vi "TAT_Start.vi"(8 "error In":errorcluster) -> (0 "error out":errorcluster)   [LabVIEW 2017]
uses:
  <vilib>/Utility/error.llb/DialogType.ctl
  Controls/Ass. Loop Control.ctl
  <vilib>/addons/database/Connection.llb/Conn ObjectReference.ctl
  2ffc4e95-467e-4723-8c12-a792954531b5.vi
  8539105e-fe5f-4c29-a376-e00596b22cdb.vi
  <vilib>/addons/database/Connection.llb/DB Tools Open Connec (Path).vi
  Global/Global 1.vi
  <vilib>/Instr/_visa.llb/VISA Configure Serial Port (Instr).vi
  <vilib>/addons/database/NI_Database_API.lvlib
  <vilib>/Utility/config.llb/NI_LVConfig.lvlib
panel:
  out "Para Value":T1
  out "PREVIOUS BARCODE":string
  out "PACKAGED QUANTITY":string
  out "SCANNED QUANTITY":string
  out "PACKAGE STICKER":string
  out "PRN to Print":string
  out "CYCLE RESULT:-":bool caption="LEAK RESULT:-"
  out "CYCLE STATUS STATION 2":string caption="CYCLE STATUS 2:-"
  out "SERIAL NO.:- 2":dbl
  in  "Model Selection:-":string(combo)
  out "CYCLE TIME:-":u32
  out "BARCODE STATION 2":string caption="QR CODE :-"
  out "CYCLE START:-":bool caption="LEAK RESULT:-"
  out "PREVIOUS BARCODE":string[](array[string])
  out "scanned":string
  out "Scanned Qty  2":string
  out "PROJECT :-":string
  out "PACKAGE Qty":string
  out "TORISHI CODE:-":string
  out "PART No.:-":string
  out "PLC STATUS:-":bool
  in  "Stop":bool
  out "QR STATION 1":string caption="QR CODE:-"
  out "RESULT STATION 1":bool caption="FINAL RESULT:-"
  out "USER:-":string
  out "PART NAME :-":string
  in  "ASS-Alarms":bool
  out "CYCLE STATUS STATION 1":string caption="CYCLE STATUS 1:-"
  out "DATE/TIME":string
  # "KAPSE SONS ROBOTICS\n& AUTOMATION"
  # "MODEL SELECTION:-"
  # "MIN"
  # "MAX"
  # "ACTUAL"
  # "STATUS"
  # "BLINKER CURRENT (mA)"
  # "POWER FOLD CURRENT (mA)"
  # "Nm"
  # "GLASS ACTUATOR CURRENT-1 (mA)"
  # "GLASS ACTUATOR CURRENT-2 (mA)"
  # "GROUND (Deg)"
  # "SKY (Deg)"
  # "EXTERIOR (Deg)"
  # "INTERIOR (Deg)"
  # "GLASS PULL OUT LOAD (Kg)"
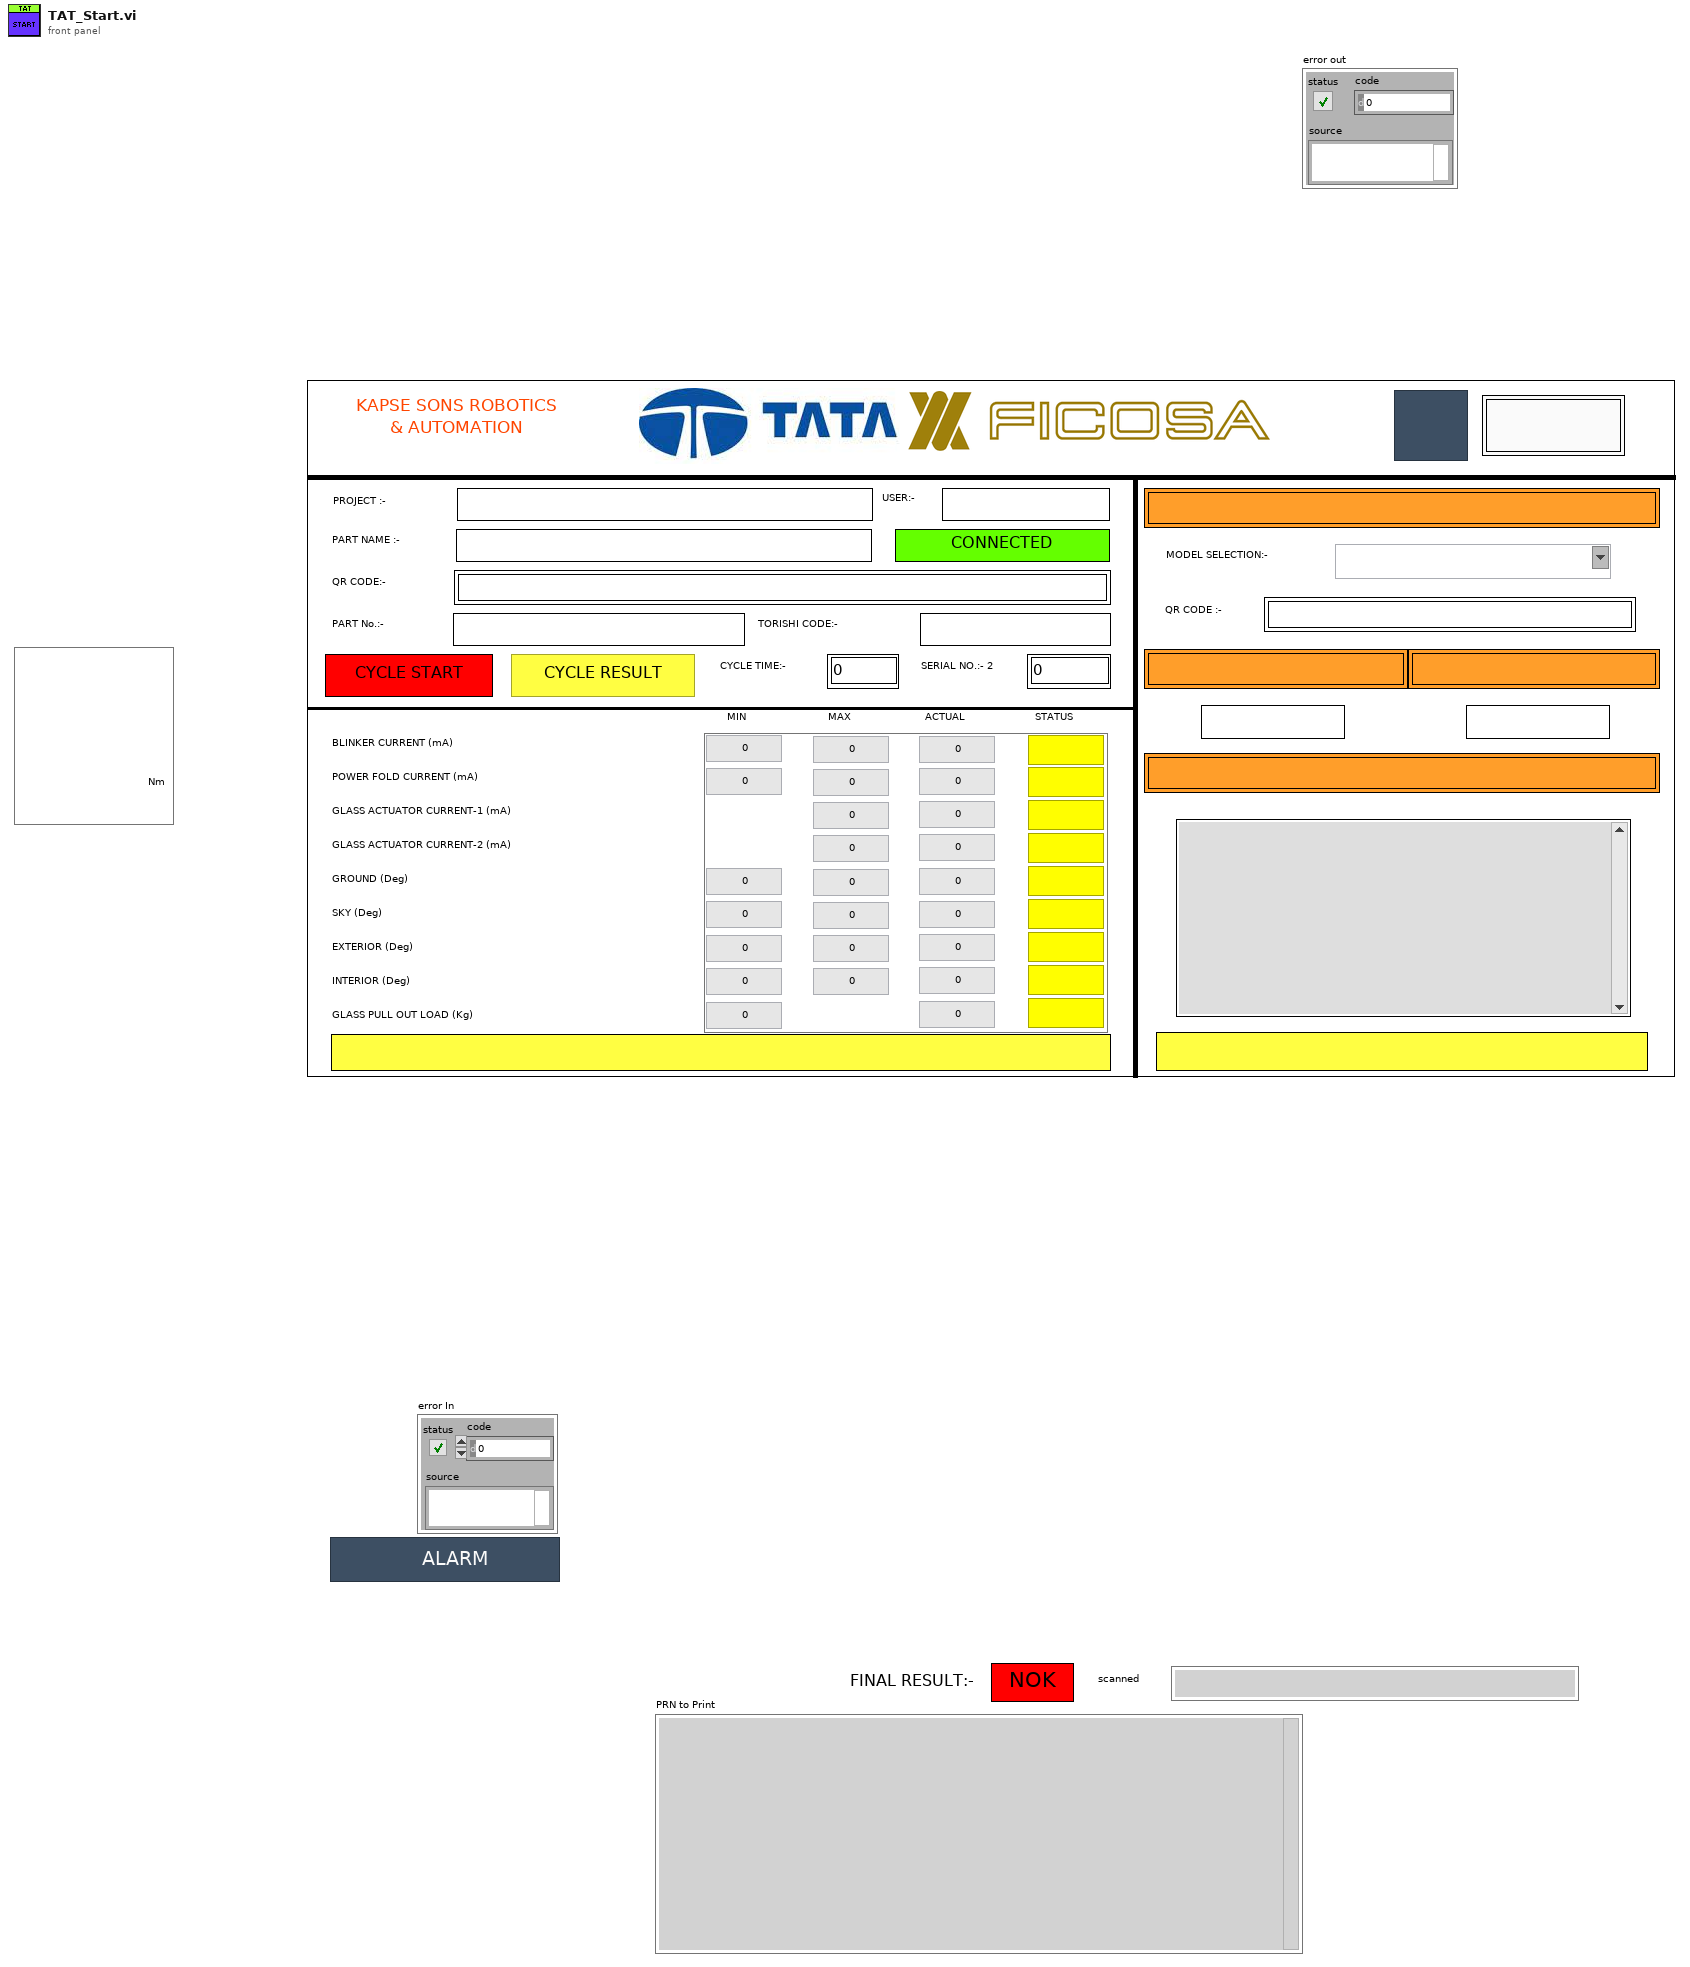
[diagram p1: front panel]
types:
  T1 = cluster{"1.1":dbl, "1.2":dbl, "1.3":dbl, "2.1":dbl, "2.2":dbl, "2.3":dbl, "3.2":dbl, "3.3":dbl, "4.2":dbl, "4.3":dbl, "5.1":dbl, "5.2":dbl, "5.3":dbl, "6.1":dbl, "6.2":dbl, "6.3":dbl, "7.1":dbl, "7.2":dbl, "7.3":dbl, "8.1":dbl, "8.2":dbl, "8.3":dbl, "9.1":dbl, "9.3":dbl, "1.4 CYCLE START":bool, "2.4 CYCLE START":bool, "3.4 CYCLE START":bool, "4.4 CYCLE START":bool, "5.4 CYCLE START":bool, "6.4 CYCLE START":bool, "7.4 CYCLE START":bool, "8.4 CYCLE START":bool, "9.4 CYCLE START":bool}
  T2 = typedef "NI_Database_API.lvlib/Conn ObjectReference.ctl" = refnum<k1>
  T3 = cluster{"Varient number":u16, "Part name":string, "connection reference":T2, "Batch_Size":u16, "PART_NO":string, "TORISHI_CODE":string, "scanner com":refnum<visa-resource-name>, "Part Name List":string[], "Varient path":path, "Current Varient path":path, "Communication path":path, "Package path":path, "Part PRN path":path, "Station2 printer IP":string, "Station1 printer IP":string, "Current Serial Number":string, "Station1_QR":string, "Serial_Number":path, "PRIVIOUS code":string[], "Barcode station 2 to log Dn":string, "Barcode station 2 to log Up":string}
  T4 = cluster{"Varient number":u16, "Part name":string, "Barcode":string, "connection reference":T2, "Batch_Size":u16, "PART_NO":string, "TORISHI_CODE":string, "scanner com":refnum<visa-resource-name>, "Part Name List":string[], "Varient path":path, "Current Varient path":path, "Communication path":path, "Package path":path, "Part PRN path":path, "Station2 printer IP":string, "Station1 printer IP":string, "Current Serial Number":string, "Station1_QR":string, "Serial_Number":path, "PRIVIOUS code":string[], "Barcode station 2 to log":string}
  T5 = typedef "Ass. Loop Control.ctl" = enum16{"Package_Qty_Count", "GENERATE_QR_PRNT", "Cluster_update", "Waiting_for_scan", "barcode CHECK", "Int", "SaveReport ", "Barcode Print", "Start Cycle", "Wait", "Cycle End", "Stop"}
  T6 = typedef "DialogType.ctl" = u16
  T7 = enum32{"invalid app kind", "Development System", "Run Time System", "Student Edition", "Embedded LabVIEW", "Evaluation", "Custom"}
  T8 = typedef "NI_LVConfig.lvlib/Config Data RefNum.ctl" = refnum<k1>
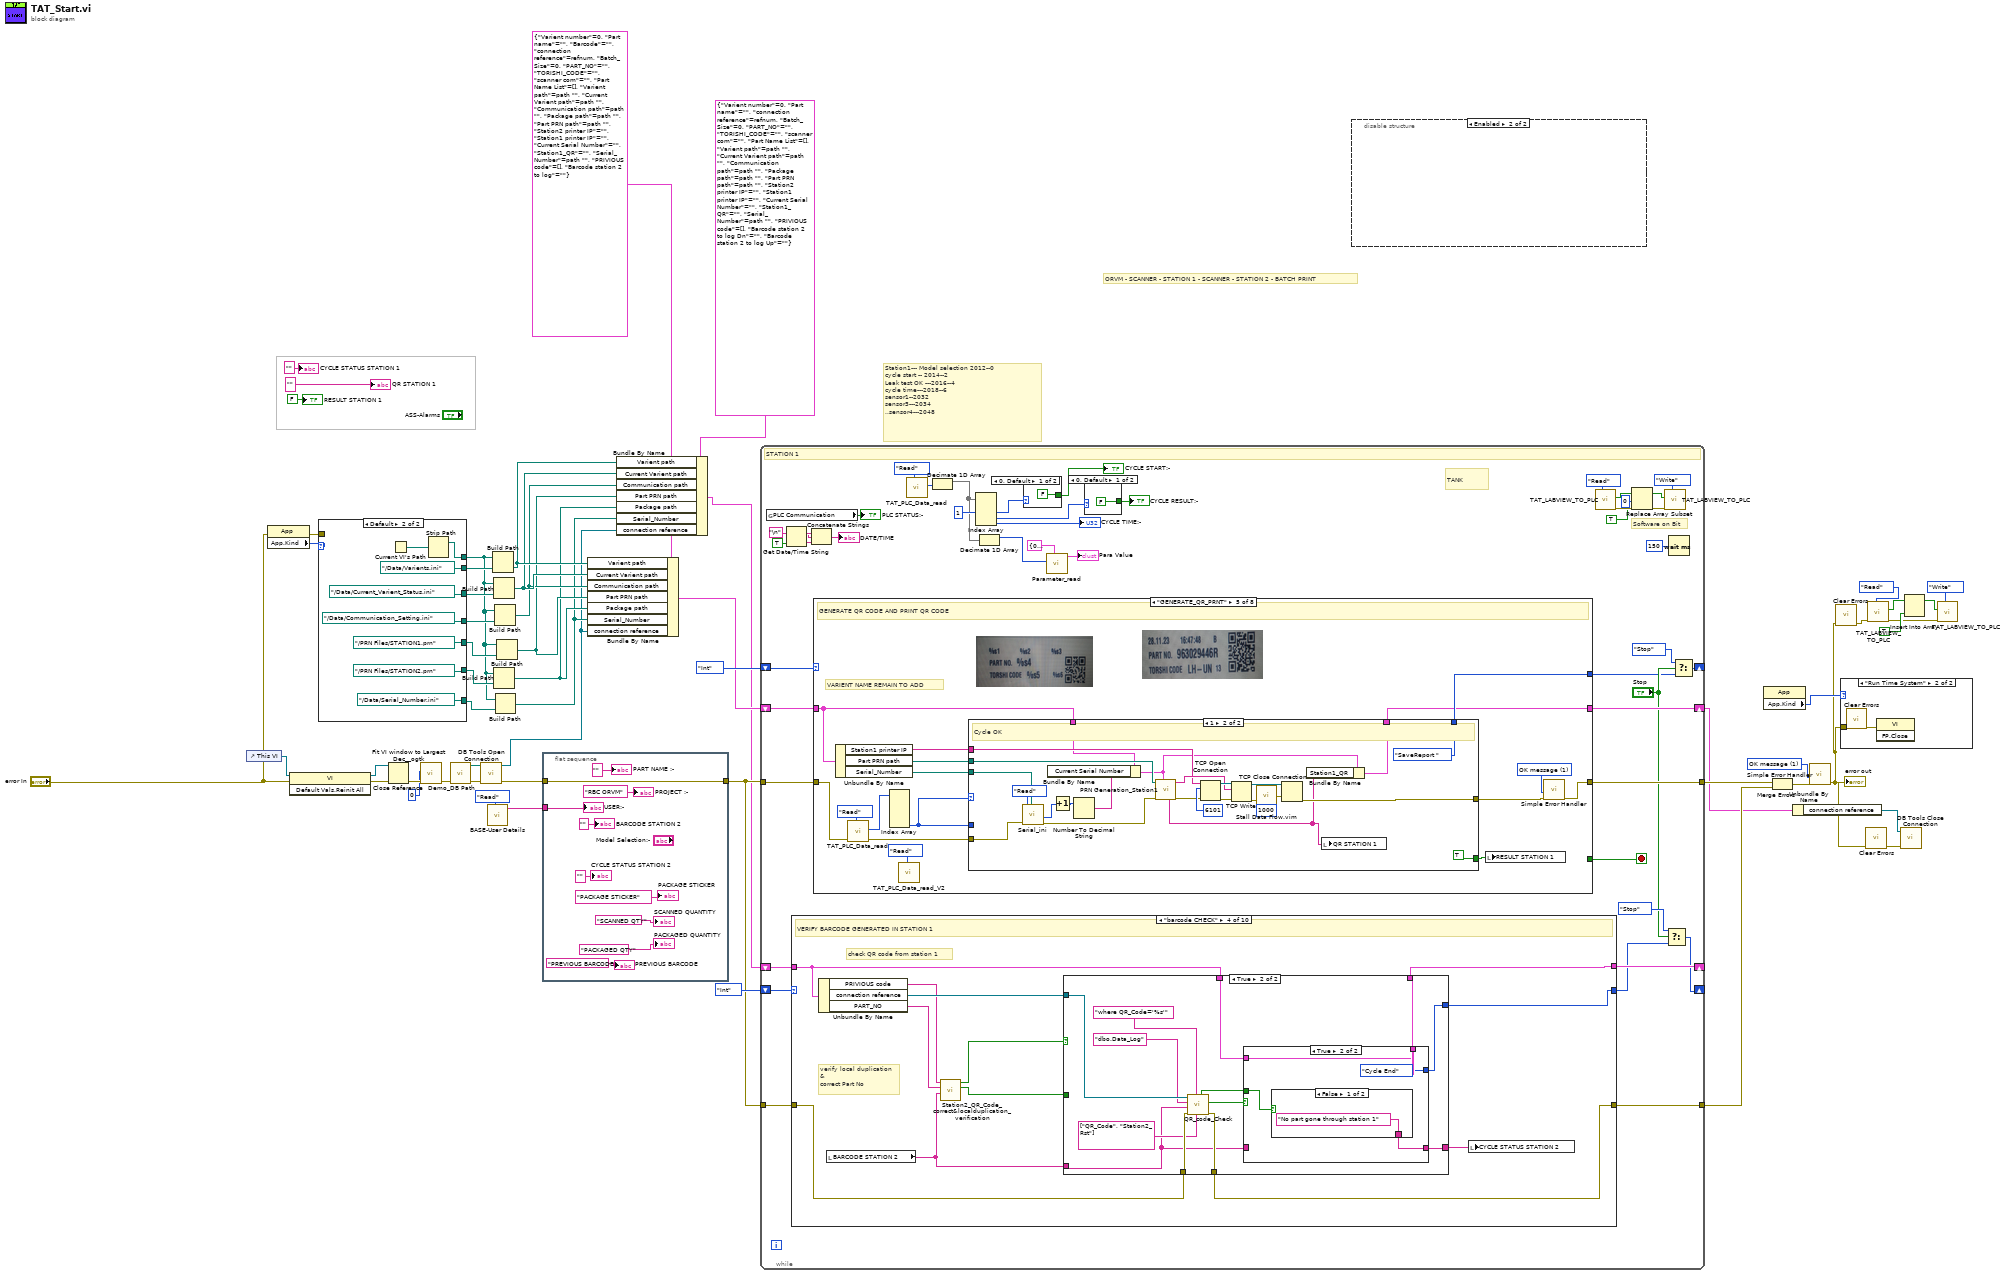
[diagram p0: block diagram]
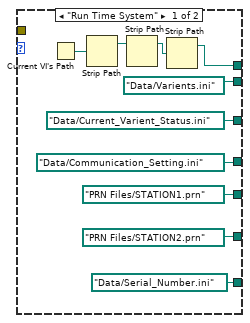
[diagram p2: hidden frame]
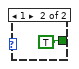
[diagram p5: hidden frame]
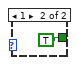
[diagram p6: hidden frame]
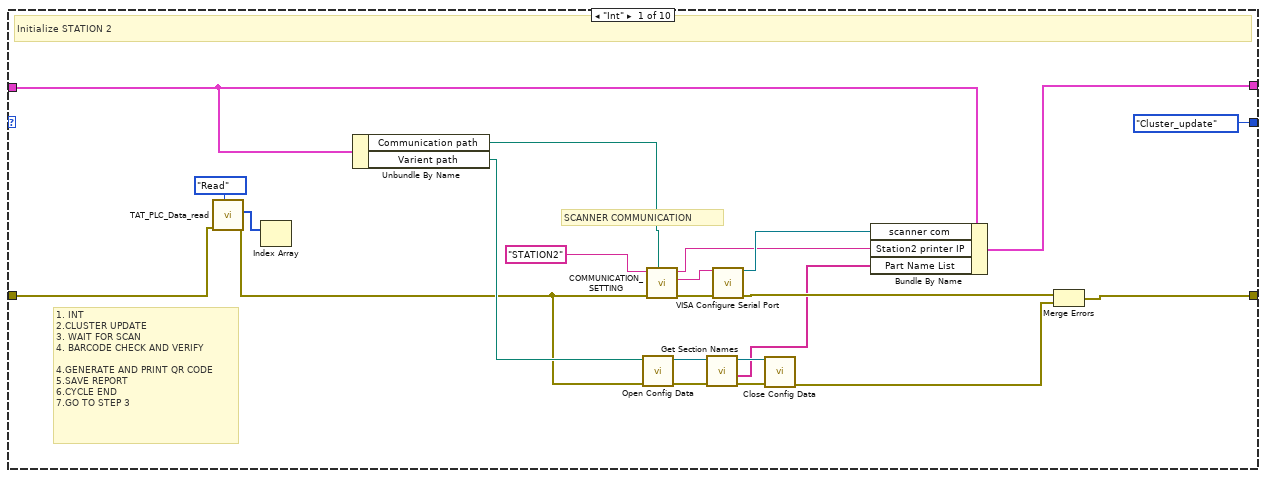
[diagram p7: hidden frame]
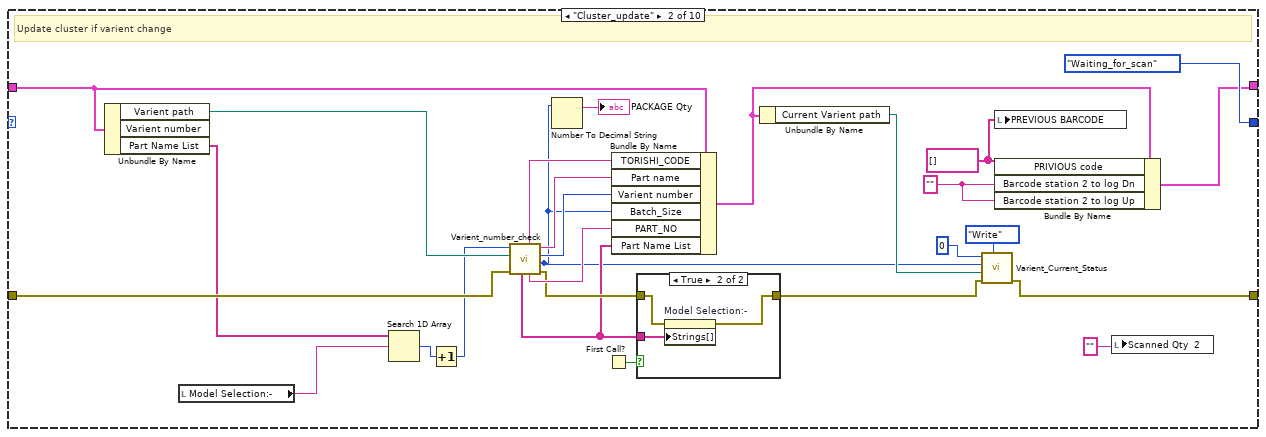
[diagram p8: hidden frame]
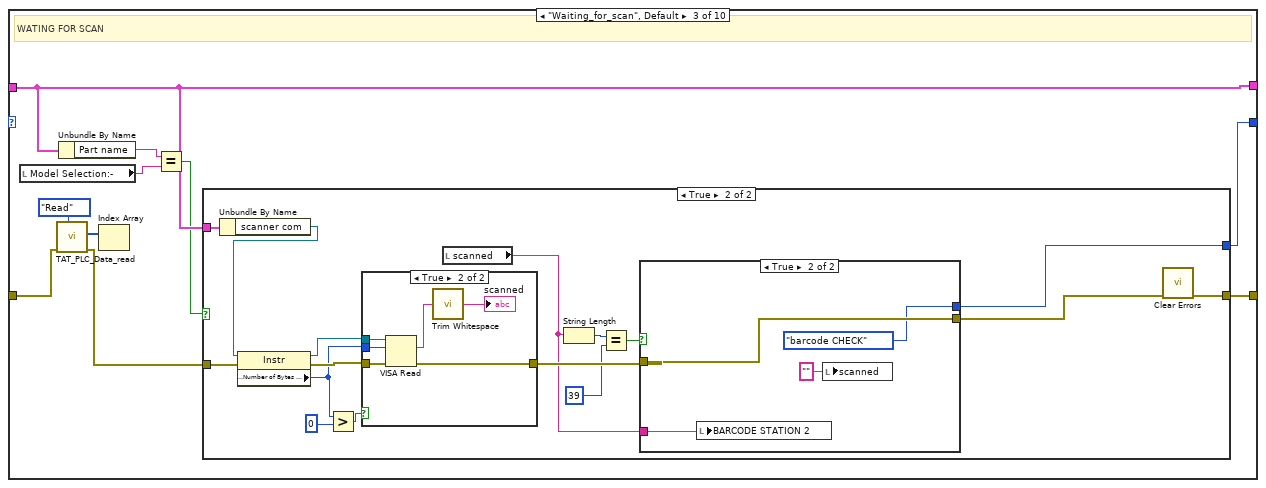
[diagram p10: hidden frame]
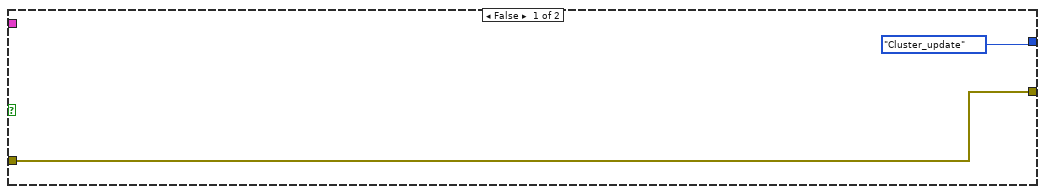
[diagram p11: hidden frame]
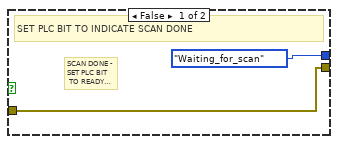
[diagram p13: hidden frame]
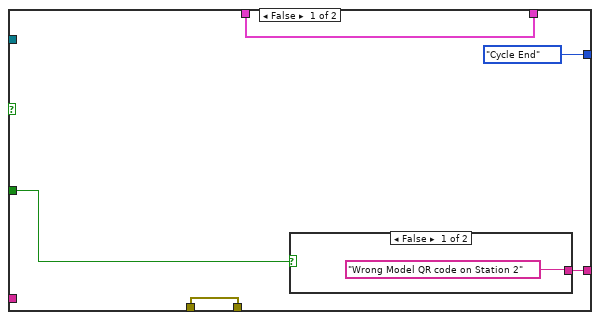
[diagram p14: hidden frame]
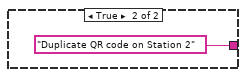
[diagram p15: hidden frame]
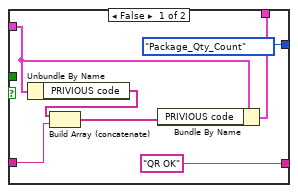
[diagram p16: hidden frame]
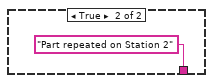
[diagram p17: hidden frame]
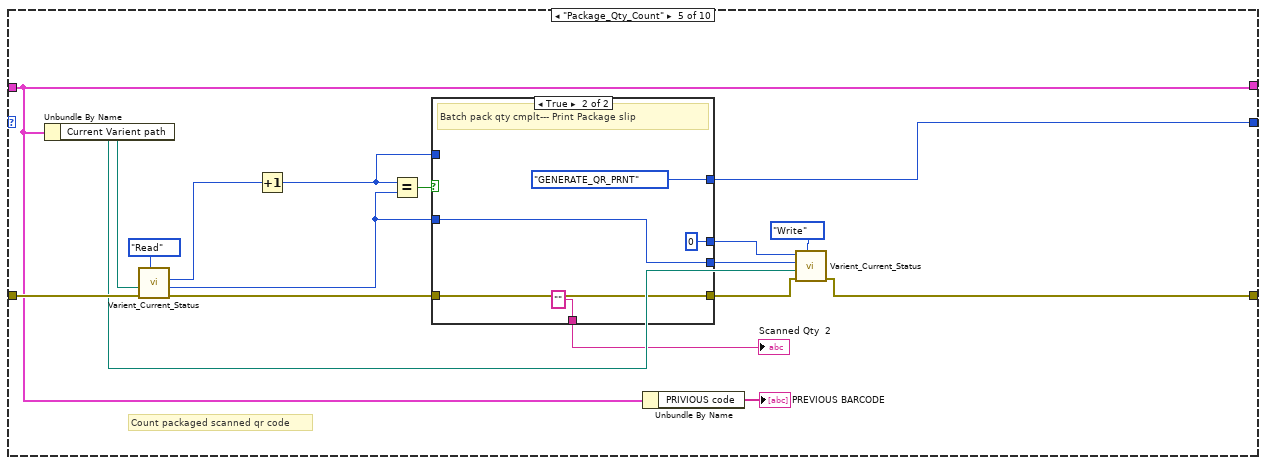
[diagram p18: hidden frame]
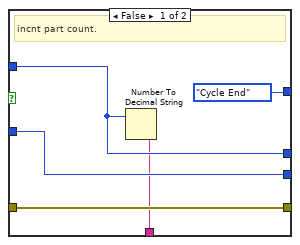
[diagram p19: hidden frame]
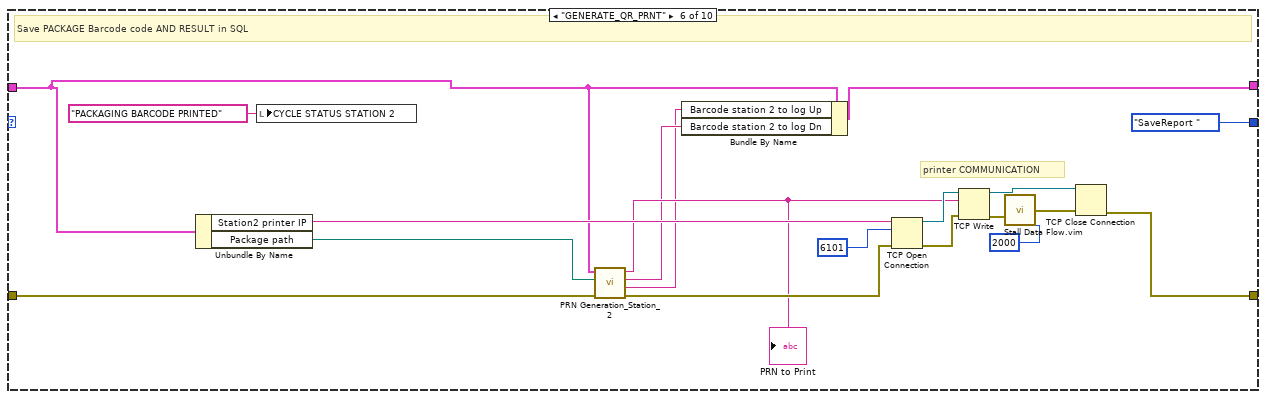
[diagram p20: hidden frame]
diagram:
  w42 = T6 1 items=["no dialog", "OK message", "continue or stop message", "OK message + warnings", "continue/stop + warnings"] ("type of dialog (OK msg:1)")
  # "Station1--- Model selection 2012--0\ncycle start -- 2014--2\nLeak test OK ---2016--4\ncycle time---2018--6\nsensor1--2032\nsensor3---2034\n..sensor4---2048"
  # "ORVM - SCANNER - STATION 1 - SCANNER - STATION 2 - BATCH PRINT"
  n1 = control-ref of="This VI"() -> (w54:refnum<vi>)
  n2 = property class="App"(error in="error In") -> (error out=w32:errorcluster, "App.Kind"=w37:T7)  [unwired: 1 in, 1 out]
  n3 = invoke class="VI" method="Default Vals.Reinit All"(reference=w54, error in="error In") -> (reference out=w52:refnum<vi>, error out=w53:errorcluster)  [unwired: 1 in, 1 out]
  n4 = case shown="Default" w37 {
    tunnel: [path "Data/Varients.ini" ("path") path "../Data/Varients.ini" ("path")] -> w36
    tunnel: [w60 w70] -> w27
    tunnel: [path "Data/Current_Varient_Status.ini" ("path") path "../Data/Current_Varient_Status.ini" ("path")] -> w35
    tunnel: [path "Data/Communication_Setting.ini" ("path") path "../Data/Communication_Setting.ini" ("path")] -> w34
    tunnel: [path "PRN Files/STATION2.prn" ("path") path "../PRN Files/STATION2.prn" ("path")] -> w33
    tunnel: w32 -> [_ _]
    tunnel: [path "PRN Files/STATION1.prn" ("path") path "../PRN Files/STATION1.prn" ("path")] -> w30
    tunnel: [path "Data/Serial_Number.ini" ("path") path "../Data/Serial_Number.ini" ("path")] -> w26
    frame "Run Time System" {
      n5 = Current VI's Path() -> (path=w63:path)
      n6 = Strip Path(path=w63) -> (stripped path=w62:path)  [unwired: 1 out]
      n7 = Strip Path(path=w62) -> (stripped path=w61:path)  [unwired: 1 out]
      n8 = Strip Path(path=w61) -> (stripped path=w60:path)  [unwired: 1 out]
    }
    frame Default {
      n9 = Current VI's Path() -> (path=w71:path)
      n10 = Strip Path(path=w71) -> (stripped path=w70:path)  [unwired: 1 out]
    }
  }
  n11 = Close Reference(reference=w52, error in (no error)=w53) -> (error out=w51:errorcluster)
  n12 = call <userlib>:"Fit VI window to Largest Dec__ogtk.vi"("error in (no error)"=w51, "border spacing (2 px)"=0) -> ("error out"=w16:errorcluster)  [unwired: 4 in, 1 out]
  n13 = call "Demo_DB Path.vi"("error in"=w16) -> ("error out"=w18:errorcluster, "DB Path"=w17:path)  [unwired: 9 in]
  n14 = call-poly <vilib>:"DB Tools Open Connection.vi"("error in (no error)"=w18, "connection information"=w17) -> ("error out"=w15:errorcluster, "connection reference"=w4:T2)  [unwired: 6 in]
  n15 = call "BASE-User Details.vi"("Enum"=enum16{"Read", "Write"}."Read") -> ("User Name Out"=w43:string)  [unwired: 9 in, 1 out]
  n16 = Build Path(base path=w27, name or relative path=w36) -> (appended path=w10:path)
  n17 = Build Path(base path=w27, name or relative path=w35) -> (appended path=w9:path)
  n18 = Build Path(base path=w27, name or relative path=w33) -> (appended path=w6:path)
  n19 = Build Path(base path=w27, name or relative path=w34) -> (appended path=w8:path)
  n20 = Build Path(base path=w27, name or relative path=w26) -> (appended path=w5:path)
  n21 = Build Path(base path=w27, name or relative path=w30) -> (appended path=w7:path)
  n22 = flat-sequence {
    tunnel: [w82] -> w40
    tunnel: w15 -> [w82]
    tunnel: w43 -> [w80]
    frame #0 {
      "USER:-" <- w80
      "PART NAME :-" <- ""
      "PROJECT :-" <- "RBC ORVM" ("PROJECT")
      "BARCODE STATION 2" <- "" ("BARCODE STATION 2")
      "CYCLE STATUS STATION 2" <- "" ("CYCLE STATUS STATION 2")
      "PACKAGE STICKER" <- "PACKAGE STICKER" ("PACKAGE STICKER")
      "SCANNED QUANTITY" <- "SCANNED QTY" ("PACKAGE STICKER")
      "PACKAGED QUANTITY" <- "PACKAGED QTY" ("PACKAGE STICKER")
      "PREVIOUS BARCODE" <- "PREVIOUS BARCODE" ("PACKAGE STICKER")
    }
  }
  n23 = Bundle By Name(cluster=T4 {"Varient number"=0, "Part name"="", "Barcode"="", "connection reference"=refnum, "Batch_Size"=0, "PART_NO"="", "TORISHI_CODE"="", "scanner com"="", "Part Name List"=[], "Varient path"=path "", "Current Varient path"=path "", "Communication path"=path "", "Package path"=path "", "Part PRN path"=path "", "Station2 printer IP"="", "Station1 printer IP"="", "Current Serial Number"="", "Station1_QR"="", "Serial_Number"=path "", "PRIVIOUS code"=[], "Barcode station 2 to log"=""}, "Varient path"=w10, "Current Varient path"=w9, "Communication path"=w8, "Part PRN path"=w7, "Package path"=w6, "Serial_Number"=w5, "connection reference"=w4) -> (w28:T4)
  n24 = Bundle By Name(cluster=T3 {"Varient number"=0, "Part name"="", "connection reference"=refnum, "Batch_Size"=0, "PART_NO"="", "TORISHI_CODE"="", "scanner com"="", "Part Name List"=[], "Varient path"=path "", "Current Varient path"=path "", "Communication path"=path "", "Package path"=path "", "Part PRN path"=path "", "Station2 printer IP"="", "Station1 printer IP"="", "Current Serial Number"="", "Station1_QR"="", "Serial_Number"=path "", "PRIVIOUS code"=[], "Barcode station 2 to log Dn"="", "Barcode station 2 to log Up"=""}, "Varient path"=w10, "Current Varient path"=w9, "Communication path"=w8, "Part PRN path"=w7, "Package path"=w6, "Serial_Number"=w5, "connection reference"=w4) -> (w2:T3)
  n25 = while {
    tunnel: w40 -> [w121]
    shift-right: [w120] -> _
    shift-left: Ass._Loop_Control."Int" ("Enum") -> [w126]
    shift-right: [w124] -> w11
    shift-left: w28 -> [w123]
    tunnel: [w122] -> w47
    shift-right: [w106] -> _
    shift-left: Ass._Loop_Control."Int" ("Enum") -> [w112]
    tunnel: w40 -> [w111]
    shift-right: [w109] -> _
    shift-left: w2 -> [w110]
    tunnel: [w108] -> w39
    stop <- w113 stop-if-true
    # "Software on Bit"
    # "TANK"
    # "STATION 1"
    n26 = global read "Global 1.vi" "PLC Communication"() -> (→"PLC STATUS:-":bool)
    n27 = Get Date/Time String(want seconds? (F)=TRUE) -> (date string=w117:string, time string=w116:string)  [unwired: 2 in]
    n28 = case shown="\"barcode CHECK\"" w112 {
      tunnel: [Ass._Loop_Control."Cluster_update" ("Enum") Ass._Loop_Control."Waiting_for_scan" ("Enum") w192 w229 w274 Ass._Loop_Control."SaveReport " ("Enum") Ass._Loop_Control."Cycle End" ("Enum") Ass._Loop_Control."Waiting_for_scan" ("Enum") Ass._Loop_Control."Stop" ("Enum") Ass._Loop_Control."Wait" ("Enum")] -> w105
      tunnel: [w149 w155 w187 w235 w273 w299 w320 w323 w328 w332] -> w109
      tunnel: [w137 w161 w193 w233 w280 w306 w319 w324 w329 w333] -> w108
      tunnel: w111 -> [w132 w178 w189 w234 w286 w304 w321 w324 w326 w333]
      tunnel: w110 -> [w145 w171 w187 w236 w273 w300 w318 w323 w328 w332]
      frame "Int" {
        # "1. INT\n2.CLUSTER UPDATE\n3. WAIT FOR SCAN\n4. BARCODE CHECK AND VERIFY\n\n4.GENERATE AND PRINT QR CODE\n5.SAVE REPORT\n6.CYCLE END\n7.GO TO STEP 3"
        # "SCANNER COMMUNICATION"
        # "Initialize STATION 2"
        n29 = call "TAT_PLC_Data_read.vi"("Enum"=enum16{"Read", "Write"}."Read", "error in (no error)"=w132) -> ("error out"=w131:errorcluster, "Array 2"=w134:u16[])  [unwired: 8 in]
        n30 = Index Array(array=w134) -> ()  [unwired: 1 in, 1 out]
        n31 = Unbundle By Name(w145) -> ("Communication path"=w144:path, "Varient path"=w135:path)
        n32 = call <vilib>:"Open Config Data.vi"("error in (no error)"=w131, "configuration file path"=w135) -> ("error out"=w142:errorcluster, "refnum"=w143:T8)  [unwired: 7 in, 1 out]
        n33 = call "COMMUNICATION_SETTING.vi"("communication path"=w144, "error in"=w131, "STATION"="STATION2") -> ("error out"=w151:errorcluster, "SCAN_COM"=w147:string, "PRINT_COM"=w146:string)  [unwired: 6 in]
        n34 = call <vilib>:"Get Section Names.vi"("error in (no error)"=w142, "refnum"=w143) -> ("error out"=w141:errorcluster, "section names"=w136:string[], "refnum out"=w140:T8)  [unwired: 7 in]
        n35 = call-poly "VISA Configure Serial Port"("VISA resource name"=w147, "error in (no error)"=w151) -> ("VISA resource name out"=w148:refnum<visa-resource-name>, "error out"=w138:errorcluster)  [unwired: 12 in]
        n36 = call <vilib>:"Close Config Data.vi"("error in (no error)"=w141, "refnum"=w140) -> ("error out"=w139:errorcluster)  [unwired: 8 in, 1 out]
        n37 = Bundle By Name(cluster=w145, "scanner com"=w148, "Station2 printer IP"=w146, "Part Name List"=w136) -> (w149:T3)
        n38 = Merge Errors(w138, w139) -> (w137:errorcluster)
      }
      frame "Cluster_update" {
        w153 = "" ("Barcode station 2 to log")
        w154 = string[] [] ("PREVIOUS Code")
        # "Update cluster if varient change"
        n39 = Unbundle By Name(w171) -> ("Varient path"=w177:path, "Part Name List"=w168:string[])  [unwired: 1 out]
        n40 = local read "Model Selection:-"() -> (w166:string)
        n41 = Search 1D Array(1D array=w168, element=w166) -> (index of element=w170:i32)  [unwired: 1 in]
        n42 = Increment(x=w170) -> (x+1=w167:i32)
        n43 = call "Varient_number_check.vi"("error in"=w178, "Varient path"=w177, "Varient No."=w167) -> ("error out"=w172:errorcluster, "Batch Size"=w159:i32, "Varient Number"=w164:i32, "Part Name"=w175:string, "PART_NO"=w174:string, "TORISHI_CODE"=w176:string, "MODEL LIST"=w169:string[])  [unwired: 2 in]
        n44 = Number To Decimal String(number=w159) -> (decimal integer string=→"PACKAGE Qty":string)  [unwired: 1 in]
        n45 = First Call?() -> (First Call?: T/F=w165:bool)
        n46 = Bundle By Name(cluster=w171, "TORISHI_CODE"=w176, "Part name"=w175, "Varient number"=w164, "Batch_Size"=w159, "PART_NO"=w174, "Part Name List"=w169) -> (w156:T3)
        n47 = case shown="True" w165 {
          tunnel: w172 -> [w180 w183]
          tunnel: [w180 w182] -> w162
          tunnel: w169 -> [_ w181]
          frame False {
          }
          frame True {
            n48 = property on="Model Selection:-" class="CmbBox"(error in=w183, "Strings[]"=w181) -> (error out=w182:errorcluster)  [unwired: 1 in, 1 out]
          }
        }
        n49 = Unbundle By Name(w156) -> ("Current Varient path"=w160:path)
        n50 = call "Varient_Current_Status.vi"("Enum"=enum16{"Write", "Read"}."Write", "error in"=w162, "Current Varient Status"=w160, "Batch Size"=w159, "Varient count"=0) -> ("error out"=w161:errorcluster)  [unwired: 4 in, 2 out]
        n51 = local write "PREVIOUS BARCODE"(w154) -> ()
        n52 = Bundle By Name(cluster=w156, "PRIVIOUS code"=w154, "Barcode station 2 to log Dn"=w153, "Barcode station 2 to log Up"=w153) -> (w155:T3)
        n53 = local write "Scanned Qty  2"("") -> ()
      }
      frame "Waiting_for_scan", Default {
        # "WATING FOR SCAN"
        n54 = local read "Model Selection:-"() -> (w185:string)
        n55 = call "TAT_PLC_Data_read.vi"("Enum"=enum16{"Read", "Write"}."Read", "error in (no error)"=w189) -> ("error out"=w188:errorcluster, "Array 2"=w191:u16[])  [unwired: 8 in]
        n56 = Unbundle By Name(w187) -> ("Part name"=w186:string)
        n57 = Index Array(array=w191) -> ()  [unwired: 1 in, 1 out]
        n58 = Equal?(x=w186, y=w185) -> (x = y?=w184:bool)
        n59 = case shown="True" w184 {
          tunnel: [w195 w211] -> w193
          tunnel: [Ass._Loop_Control."Cluster_update" ("Enum") w206] -> w192
          tunnel: w188 -> [w195 w205]
          tunnel: w187 -> [_ w204]
          frame False {
          }
          frame True {
            n60 = Unbundle By Name(w204) -> ("scanner com"=w203:refnum<visa-resource-name>)
            n61 = property class="Instr"(reference=w203, error in=w205) -> (reference out=w210:refnum<visa-resource-name>, error out=w209:errorcluster, "Serial Settings:Number of Bytes at Serial Port"=w196:u32)
            n62 = Greater?(x=w196, y=u32 0) -> (0:w197:bool)
            n63 = case shown="True" w197 {
              tunnel: w210 -> [_ w218]
              tunnel: w209 -> [w212 w217]
              tunnel: w196 -> [_ w216]
              tunnel: [w212 w215] -> w208
              frame False {
              }
              frame True {
                n64 = VISA Read(VISA resource name=w218, byte count=w216, error in (no error)=w217) -> (read buffer=w214:string, error out=w215:errorcluster)  [unwired: 2 out]
                n65 = call <vilib>:"Trim Whitespace.vi"("string"=w214) -> ("trimmed string"=→"scanned":string)  [unwired: 1 in]
              }
            }
            n66 = local read "scanned"() -> (w200:string)
            n67 = String Length(string=w200) -> (length=w202:i32)
            n68 = Equal?(x=w202, y=39) -> (x = y?=w199:bool)
            n69 = case shown="True" w199 {
              tunnel: w208 -> [w220 w224]
              tunnel: [w220 w224] -> w207
              tunnel: w200 -> [_ w221]
              tunnel: [Ass._Loop_Control."Waiting_for_scan" ("Enum") Ass._Loop_Control."barcode CHECK" ("Enum")] -> w206
              frame False {
                # "SCAN DONE - SET PLC BIT\n TO READY CYCLE"
                # "SET PLC BIT TO INDICATE SCAN DONE"
              }
              frame True {
                n70 = local write "BARCODE STATION 2"(w221) -> ()
                n71 = local write "scanned"("" ("scanned")) -> ()
              }
            }
            n72 = call <vilib>:"Clear Errors.vi"("error in (no error)"=w207) -> ("error out"=w211:errorcluster)  [unwired: 5 in, 1 out]
          }
        }
      }
      frame "barcode CHECK" {
        # "verify local duplication\n&\ncorrect Part No"
        # "check QR code from station 1"
        # "VERIFY BARCODE GENERATED IN STATION 1"
        n73 = Unbundle By Name(w236) -> ("PRIVIOUS code"=w228:string[], "connection reference"=w232:T2, "PART_NO"=w231:string)
        n74 = local read "BARCODE STATION 2"() -> (w227:string)
        n75 = call "Station2_QR_Code_correct&localduplication_verification.vi"("BARCODE STATION in"=w227, "PART_NO"=w231, "PRIVIOUS code"=w228) -> ("Correct part no True"=w225:bool, "Correct part no & No duplication TRUE"=w226:bool)  [unwired: 7 in]
        n76 = case shown="True" w226 {
          tunnel: w236 -> [w241 w256]
          tunnel: [w241 w255] -> w235
          tunnel: w234 -> [w240 w254]
          tunnel: [w240 w253] -> w233
          tunnel: w232 -> [_ w252]
          tunnel: w227 -> [_ w247]
          tunnel: [w239 w249] -> w230
          tunnel: [Ass._Loop_Control."Cycle End" ("Enum") w248] -> w229
          tunnel: w225 -> [w237 _]
          frame False {
            n77 = case shown="False" w237 {
              tunnel: ["Wrong Model QR code on Station 2" ("Cycle Status") "Duplicate QR code on Station 2" ("Cycle Status")] -> w239
              frame False {
              }
              frame True {
              }
            }
          }
          frame True {
            n78 = call "QR_code_Check.vi"("Columns"=string[] ["QR_Code", "Station2_Rst"] ("columns 2"), "format string"="where QR_Code='%s'", "error in (no error)"=w254, "replace %s"=w247, "table"="dbo.Data_Log", "Refnum in"=w252) -> ("error out"=w253:errorcluster, "FALSE healty"=w245:bool, "TRUE Duplication on Station 2"=w244:bool)  [unwired: 2 out]
            n79 = case shown="True" w245 {
              tunnel: ["QR OK" ("Cycle Status") w267] -> w249
              tunnel: w256 -> [w260 w266]
              tunnel: [w262 w266] -> w255
              tunnel: [Ass._Loop_Control."Package_Qty_Count" ("Enum") Ass._Loop_Control."Cycle End" ("Enum")] -> w248
              tunnel: w247 -> [w257 _]
              tunnel: w244 -> [_ w264]
              frame False {
                n80 = Unbundle By Name(w260) -> ("PRIVIOUS code"=w259:string[])
                n81 = Build Array (concatenate)(w259, w257) -> (w258:string[])
                n82 = Bundle By Name(cluster=w260, "PRIVIOUS code"=w258) -> (w262:T3)
              }
              frame True {
                n83 = case shown="False" w264 {
                  tunnel: ["No part gone through station 1" ("Cycle Status") "Part repeated on Station 2" ("Cycle Status")] -> w267
                  frame False {
                  }
                  frame True {
                  }
                }
              }
            }
          }
        }
        n84 = local write "CYCLE STATUS STATION 2"(w230) -> ()
      }
      frame "Package_Qty_Count" {
        # "Count packaged scanned qr code"
        n85 = Unbundle By Name(w273) -> ("Current Varient path"=w272:path)
        n86 = call "Varient_Current_Status.vi"("Enum"=enum16{"Write", "Read"}."Read", "error in"=w286, "Current Varient Status"=w272) -> ("error out"=w284:errorcluster, "Batch Size"=w277:i32, "Varient Count"=w283:i32)  [unwired: 6 in]
        n87 = Increment(x=w283) -> (x+1=w278:i32)
        n88 = Equal?(x=w278, y=w277) -> (x = y?=w282:bool)
        n89 = case shown="True" w282 {
          tunnel: [w291 w296] -> w279
          tunnel: w284 -> [w291 w296]
          tunnel: w278 -> [w288 _]
          tunnel: w277 -> [w290 w295]
          tunnel: [w290 w295] -> w276
          tunnel: [w288 0] -> w275
          tunnel: [Ass._Loop_Control."Cycle End" ("Enum") Ass._Loop_Control."GENERATE_QR_PRNT" ("Enum")] -> w274
          tunnel: [w287 "" ("String")] -> w271
          frame False {
            # "incnt part count."
            n90 = Number To Decimal String(number=w288) -> (decimal integer string=w287:string)  [unwired: 1 in]
          }
          frame True {
            # "Batch pack qty cmplt--- Print Package slip"
          }
        }
        "Scanned Qty  2" <- w271
        n91 = Unbundle By Name(w273) -> ("PRIVIOUS code"=→"PREVIOUS BARCODE":string[])
        n92 = call "Varient_Current_Status.vi"("Enum"=enum16{"Write", "Read"}."Write", "error in"=w279, "Current Varient Status"=w272, "Batch Size"=w276, "Varient count"=w275) -> ("error out"=w280:errorcluster)  [unwired: 4 in, 2 out]
      }
      frame "GENERATE_QR_PRNT" {
        # "printer COMMUNICATION"
        # "Save PACKAGE Barcode code AND RESULT in SQL"
        n93 = Unbundle By Name(w300) -> ("Station2 printer IP"=w305:string, "Package path"=w302:path)
        n94 = local write "CYCLE STATUS STATION 2"("PACKAGING BARCODE PRINTED" ("Cycle Status")) -> ()
        n95 = call "PRN Generation_Station_2.vi"("error in (no error)"=w304, "PRN path"=w302, "Cluster"=w300) -> ("error out"=w303:errorcluster, "Barcode Station 2 Up"=w297:string, "Barcode station 2 Dn"=w298:string, "PRN to Print"=w301:string)  [unwired: 5 in]
        "PRN to Print" <- w301
        n96 = Bundle By Name(cluster=w300, "Barcode station 2 to log Up"=w297, "Barcode station 2 to log Dn"=w298) -> (w299:T3)
        n97 = TCP Open Connection(address=w305, remote port or service name=u16 6101, error in (no error)=w303) -> (connection ID=w311:refnum<k5>, error out=w312:errorcluster)  [unwired: 2 in]
        n98 = TCP Write(connection ID=w311, data in=w301, error in (no error)=w312) -> (connection ID out=w309:refnum<k5>, error out=w313:errorcluster)  [unwired: 1 in, 1 out]
        n99 = call "Stall Data Flow.vim"("value in"=w313, "milliseconds to wait"=u32 2000) -> ("value out"=w310:errorcluster)  [unwired: 1 out]
        n100 = TCP Close Connection(connection ID=w309, error in (no error)=w310) -> (error out=w306:errorcluster)  [unwired: 1 in, 1 out]
      }
      frame "SaveReport " {
        w316 = "" ("Barcode station 2 to log")
        w317 = string[] [] ("PREVIOUS Code")
        # "Save Barcode code AND RESULT in SQL"
        n101 = call "Station2_Data_Log.vi"("error in (no error)"=w321, "Cluster"=w318) -> ("error out"=w319:errorcluster)  [unwired: 9 in]
        n102 = Bundle By Name(cluster=w318, "PRIVIOUS code"=w317, "Barcode station 2 to log Dn"=w316, "PRIVIOUS code"=w317, "Barcode station 2 to log Up"=w316) -> (w320:T3)
        n103 = local write "PREVIOUS BARCODE"(w317) -> ()
      }
      frame "Cycle End" {
      }
      frame "Stop" {
        n104 = local write "CYCLE STATUS STATION 2"("STATION STOP" ("Cycle Status")) -> ()
        n105 = Unbundle By Name(w328) -> ("scanner com"=w327:refnum<visa-resource-name>)
        n106 = VISA Close(VISA resource name=w327, error in (no error)=w326) -> (error out=w329:errorcluster)
      }
      frame "Start Cycle" {
        n107 = local write "CYCLE STATUS STATION 1"("Cycle started" ("Cycle Status")) -> ()
      }
    }
    n108 = Concatenate Strings(w117, "\n", w116) -> (→"DATE/TIME":string)
    n109 = case shown="\"GENERATE_QR_PRNT\"" w126 {
      tunnel: [Ass._Loop_Control."Cluster_update" ("Enum") Ass._Loop_Control."Wait" ("Enum") w372 Ass._Loop_Control."Wait" ("Enum") w400 Ass._Loop_Control."Cycle End" ("Enum") Ass._Loop_Control."Wait" ("Enum") Ass._Loop_Control."Stop" ("Enum")] -> w103
      tunnel: [w343 w351 w374 w391 w398 w446 w455 w458] -> w124
      tunnel: w123 -> [w337 w350 w374 w391 w399 w446 w455 w458]
      tunnel: [_ _ FALSE _ _ _ _ TRUE] -> w113
      tunnel: [w341 w353 w361 w388 w393 w438 w454 w456] -> w122
      tunnel: w121 -> [w336 w357 w367 w388 w404 w451 w454 w456]
      frame "Int" {
        w342 = T6 1 items=["no dialog", "OK message", "continue or stop message", "OK message + warnings", "continue/stop + warnings"] ("type of dialog (OK msg:1)")
        # "1. INT\n2.CLUSTER UPDATE\n3. WAIT\n4.GENERATE AND PRINT QR CODE\n5.SAVE REPORT\n6.CYCLE END\n7.GO TO STEP 3"
        # "Initialize"
        n110 = Unbundle By Name(w337) -> ("Communication path"=w339:path)
        n111 = local write "CYCLE STATUS STATION 1"("WAIT FOR CYCLE START" ("Cycle Status")) -> ()
        n112 = call "COMMUNICATION_SETTING.vi"("communication path"=w339, "error in"=w336, "STATION"="STATION1") -> ("error out"=w340:errorcluster, "PRINT_COM"=w338:string)  [unwired: 6 in, 1 out]
        n113 = Bundle By Name(cluster=w337, "Station1 printer IP"=w338) -> (w343:T4)
        n114 = call <vilib>:"Simple Error Handler.vi"("type of dialog (OK msg:1)"=w342, "error in (no error)"=w340) -> ("error out"=w341:errorcluster)  [unwired: 3 in, 4 out]
      }
      frame "Cluster_update" {
        # "PART NAME\nPART No.\nPACKAGE QUANTITY\nTORISHI CODE"
        # "PART NAME---\nVARIENT NAME"
        # "Update cluster if varient change"
        n115 = Unbundle By Name(w350) -> ("Varient path"=w349:path)
        n116 = call "TAT_PLC_Data_read.vi"("Enum"=enum16{"Read", "Write"}."Read", "error in (no error)"=w357) -> ("error out"=w354:errorcluster, "Array 2"=w359:u16[])  [unwired: 8 in]
        n117 = Index Array(array=w359) -> (element=w348:u16)  [unwired: 1 in]
        n118 = call "Varient_number_check.vi"("error in"=w354, "Varient path"=w349, "Varient No."=w348) -> ("error out"=w353:errorcluster, "Batch Size"=w352:i32, "Part Name"=w356:string, "PART_NO"=w355:string, "TORISHI_CODE"=w347:string)  [unwired: 2 in, 2 out]
        "PART No.:-" <- w355
        "TORISHI CODE:-" <- w347
        n119 = Bundle By Name(cluster=w350, "Part name"=w356, "Varient number"=w348, "Batch_Size"=w352, "PART_NO"=w355, "TORISHI_CODE"=w347) -> (w351:T4)
        n120 = local write "PART NAME :-"(w356) -> ()
      }
      frame "Wait", Default {
        w363 = T6 1 items=["no dialog", "OK message", "continue or stop message", "OK message + warnings", "continue/stop + warnings"] ("type of dialog (OK msg:1)")
        # "Serial logic"
        # "WAITING FORM CCYLE TO COMPLE TO PRINT QR"
        # "Wait"
        n121 = Unbundle By Name(w374) -> ("Varient number"=w373:u16, "Serial_Number"=w366:path)
        n122 = call "TAT_PLC_Data_read.vi"("Enum"=enum16{"Read", "Write"}."Read", "error in (no error)"=w367) -> ("error out"=w364:errorcluster, "Array 2"=w375:u16[])  [unwired: 8 in]
        n123 = Index Array(array=w375) -> (element #1=w377:u16, element #3=w370:u16)  [unwired: 3 in, 1 out]
        n124 = Not Equal?(x=w373, y=w377) -> (x != y?=w371:bool)
        n125 = call "Serial_Logic.vi"("error in"=w367, "Serial path"=w366) -> ("error out"=w365:errorcluster)  [unwired: 9 in]
        n126 = Equal?(x=w370, y=u16 1) -> (x = y?=w368:bool)
        n127 = Merge Errors(w364, w365) -> (w362:errorcluster)
        n128 = call <userlib>:"Boolean Trigger__ogtk.vi"("Boolean Input"=w368) -> ("Rising Edge"=w382:bool, "Falling Edge"=w380:bool)  [unwired: 1 in]
        n129 = Build Array(w382, w380, w371) -> (w381:bool[])
        n130 = Search 1D Array(1D array=w381, element=TRUE ("Boolean Input")) -> (index of element=w379:i32)  [unwired: 1 in]
        n131 = case shown="1" w379 {
          tunnel: [Ass._Loop_Control."Wait" ("Enum") Ass._Loop_Control."Start Cycle" ("Enum") Ass._Loop_Control."GENERATE_QR_PRNT" ("Enum") Ass._Loop_Control."Cluster_update" ("Enum")] -> w372
          frame -1, Default {
          }
          frame 0 {
            # "CYCYLE START BIT"
          }
          frame 1 {
            # "CYCLE END STORE RLT"
          }
          frame 2 {
            # "CLUSTER UPDATE"
          }
        }
        n132 = call <vilib>:"Simple Error Handler.vi"("type of dialog (OK msg:1)"=w363, "error in (no error)"=w362) -> ("error out"=w361:errorcluster)  [unwired: 3 in, 4 out]
      }
      frame "Start Cycle" {
        n133 = local write "CYCLE STATUS STATION 1"("Cycle started" ("Cycle Status")) -> ()
      }
      frame "GENERATE_QR_PRNT" {
        w395 = T6 1 items=["no dialog", "OK message", "continue or stop message", "OK message + warnings", "continue/stop + warnings"] ("type of dialog (OK msg:1)")
        # "VARIENT NAME REMAIN TO ADD"
        # "GENERATE QR CODE AND PRINT QR CODE"
        n134 = Unbundle By Name(w399) -> ("Station1 printer IP"=w402:string, "Part PRN path"=w407:path, "Serial_Number"=w396:path)
        n135 = call "TAT_PLC_Data_read.vi"("Enum"=enum16{"Read", "Write"}."Read", "error in (no error)"=w404) -> ("error out"=w403:errorcluster, "Array 2"=w405:u16[])  [unwired: 8 in]
        n136 = Index Array(array=w405) -> (element #5=w397:u16)  [unwired: 5 in, 4 out]
        n137 = call "TAT_PLC_Data_read_V2.vi"("Enum"=enum16{"Read", "Write"}."Read") -> ()  [unwired: 9 in, 2 out]
        n138 = case shown="1" w397 {
          tunnel: w407 -> [_ w436]
          tunnel: w403 -> [w411 w419]
          tunnel: w397 -> [_ _]
          tunnel: [w411 w427] -> w394
          tunnel: w402 -> [_ w425]
          tunnel: w399 -> [w408 w413]
          tunnel: [FALSE TRUE] -> w401
          tunnel: [Ass._Loop_Control."Wait" ("Enum") Ass._Loop_Control."SaveReport " ("Enum")] -> w400
          tunnel: [w408 w422] -> w398
          tunnel: w396 -> [_ w417]
          frame 0, Default {
            # "cycyle not ok"
          }
          frame 1 {
            # "Cycle OK"
            n139 = call "Serial_ini.vi"("error in"=w419, "Serial path"=w417, "Enum"=enum16{"Write", "Read"}."Read") -> ("error out"=w420:errorcluster, "Count"=w416:u32)  [unwired: 5 in, 2 out]
            n140 = Increment(x=w416) -> (x+1=w415:u32)
            n141 = Number To Decimal String(number=w415) -> (decimal integer string=w414:string)  [unwired: 1 in]
            n142 = Bundle By Name(cluster=w413, "Current Serial Number"=w414) -> (w412:T4)
            n143 = call "PRN Generation_Station1.vi"("Part PRN QR"=w436, "error in (no error)"=w420, "Cluster"=w412) -> ("QR Code"=w421:string, "PRN to Print"=w426:string, "error out"=w428:errorcluster)  [unwired: 5 in]
            n144 = TCP Open Connection(address=w425, remote port or service name=u16 6101, error in (no error)=w428) -> (connection ID=w431:refnum<k5>, error out=w432:errorcluster)  [unwired: 2 in]
            n145 = TCP Write(connection ID=w431, data in=w426, error in (no error)=w432) -> (connection ID out=w429:refnum<k5>, error out=w434:errorcluster)  [unwired: 1 in, 1 out]
            n146 = call "Stall Data Flow.vim"("value in"=w434, "milliseconds to wait"=u32 1000) -> ("value out"=w430:errorcluster)  [unwired: 1 out]
            n147 = TCP Close Connection(connection ID=w429, error in (no error)=w430) -> (error out=w427:errorcluster)  [unwired: 1 in, 1 out]
            n148 = Bundle By Name(cluster=w412, "Station1_QR"=w421) -> (w422:T4)
            n149 = local write "QR STATION 1"(w421) -> ()
          }
        }
        n150 = local write "RESULT STATION 1"(w401) -> ()
        n151 = call <vilib>:"Simple Error Handler.vi"("type of dialog (OK msg:1)"=w395, "error in (no error)"=w394) -> ("error out"=w393:errorcluster)  [unwired: 3 in, 4 out]
      }
      frame "SaveReport " {
        w440 = T6 1 items=["no dialog", "OK message", "continue or stop message", "OK message + warnings", "continue/stop + warnings"] ("type of dialog (OK msg:1)")
        (unwired) string[] ["Date", "Time", "Model_No", "Part_Name", "Part_No", "Torishi_Code", "Shift", "Cycle_Time", "Station1_Rst", "Packaging_Qty", "Serial_No", "QR_Code", "Station2_Rst"] ("columns 2")
        # "Save Barcode code AND RESULT in SQL"
        n152 = call "Station1_Data_Log.vi"("error in (no error)"=w451, "Cluster"=w446) -> ("error out"=w448:errorcluster)  [unwired: 8 in, 1 out]
        n153 = Unbundle By Name(w446) -> ("Serial_Number"=w445:path, "Current Serial Number"=w442:string)
        n154 = Decimal String To Number(string=w442, default (0L)=u32 0 ("default (0 I32)")) -> (number=w437:u32)  [unwired: 1 in, 1 out]
        "SERIAL NO.:- 2" <- w437
        n155 = call "Serial_ini.vi"("error in"=w448, "Serial path"=w445, "Enum"=enum16{"Write", "Read"}."Read") -> ("error out"=w449:errorcluster, "Shift"=w443:string, "Date"=w444:string)  [unwired: 5 in, 1 out]
        n156 = call "Serial_ini.vi"("error in"=w449, "Serial path"=w445, "Date"=w444, "Count"=w437, "Shift"=w443, "Enum"=enum16{"Write", "Read"}."Write") -> ("error out"=w439:errorcluster)  [unwired: 2 in, 3 out]
        n157 = call <vilib>:"Simple Error Handler.vi"("type of dialog (OK msg:1)"=w440, "error in (no error)"=w439) -> ("error out"=w438:errorcluster)  [unwired: 3 in, 4 out]
      }
      frame "Cycle End" {
      }
      frame "Stop" {
        n158 = local write "CYCLE STATUS STATION 1"("STATION STOP" ("Cycle Status")) -> ()
      }
    }
    n159 = call "TAT_PLC_Data_read.vi"("Enum"=enum16{"Read", "Write"}."Read") -> ("Array 2"=w86:u16[])  [unwired: 9 in, 1 out]
    n160 = Decimate 1D Array(w86) -> (w85:u16[])  [unwired: 1 out]
    n161 = Index Array(array=w85, index #2=1 ("index")) -> (element #2=w100:u16, element #3=w97:u16, element #4=→"CYCLE TIME:-":u16)  [unwired: 3 in, 1 out]
    n162 = Decimate 1D Array(w85) -> (w84:u16[])  [unwired: 1 out]
    n163 = case shown="0, Default" w100 {
      tunnel: [FALSE TRUE] -> w99
      frame 0, Default {
      }
      frame 1 {
      }
    }
    "CYCLE START:-" <- w99
    n164 = call "Parameter_read.vi"("Para reference"=T1 {"1.1"=0.0, "1.2"=0.0, "1.3"=0.0, "2.1"=0.0, "2.2"=0.0, "2.3"=0.0, "3.2"=0.0, "3.3"=0.0, "4.2"=0.0, "4.3"=0.0, "5.1"=0.0, "5.2"=0.0, "5.3"=0.0, "6.1"=0.0, "6.2"=0.0, "6.3"=0.0, "7.1"=0.0, "7.2"=0.0, "7.3"=0.0, "8.1"=0.0, "8.2"=0.0, "8.3"=0.0, "9.1"=0.0, "9.3"=0.0, "1.4 CYCLE START"=FALSE, "2.4 CYCLE START"=FALSE, "3.4 CYCLE START"=FALSE, "4.4 CYCLE START"=FALSE, "5.4 CYCLE START"=FALSE, "6.4 CYCLE START"=FALSE, "7.4 CYCLE START"=FALSE, "8.4 CYCLE START"=FALSE, "9.4 CYCLE START"=FALSE} ("Para Value 2"), "Array"=w84) -> ("Para out"=→"Para Value":T1)  [unwired: 9 in]
    n165 = case shown="0, Default" w97 {
      tunnel: [FALSE TRUE] -> w89
      frame 0, Default {
      }
      frame 1 {
      }
    }
    "CYCLE RESULT:-" <- w89
    n166 = call "TAT_LABVIEW_TO_PLC.vi"("Enum"=enum16{"Read", "Write"}."Read") -> ("error out"=w94:errorcluster, "Array 2"=w93:bool[])  [unwired: 9 in]
    n167 = Replace Array Subset(array=w93, new element=TRUE ("new element/subarray"), index=0) -> (w92:bool[])
    n168 = call "TAT_LABVIEW_TO_PLC.vi"("Enum"=enum16{"Read", "Write"}."Write", "error in (no error)"=w94, "Array"=w92) -> ()  [unwired: 7 in, 2 out]
    n169 = Select(t=Ass._Loop_Control."Stop" ("Enum"), s="Stop", f=w105) -> (s? t:f=w106:T5)
    n170 = Wait (ms)(milliseconds to wait=u32 150) -> ()  [unwired: 1 out]
    n171 = Select(t=Ass._Loop_Control."Stop" ("Enum"), s="Stop", f=w103) -> (s? t:f=w120:T5)
  }
  n172 = disable-structure shown="Enabled" {
    frame Disabled {
    }
    frame Enabled {
    }
  }
  n173 = property class="App"() -> ("App.Kind"=w38:T7)  [unwired: 2 in, 2 out]
  n174 = Merge Errors(w47, w39) -> (w45:errorcluster)
  n175 = Unbundle By Name(w11) -> ("connection reference"=w12:T2)
  n176 = call <vilib>:"Simple Error Handler.vi"("type of dialog (OK msg:1)"=w42, "error in (no error)"=w45) -> ("error out"=w14:errorcluster)  [unwired: 3 in, 4 out]
  "error out" <- w14
  n177 = call <vilib>:"Clear Errors.vi"("error in (no error)"=w14) -> ("error out"=w19:errorcluster)  [unwired: 5 in, 1 out]
  n178 = case shown="\"Run Time System\"" w38 {
    tunnel: w14 -> [_ w462]
    frame "invalid app kind", Default {
    }
    frame "Run Time System" {
      n179 = call <vilib>:"Clear Errors.vi"("error in (no error)"=w462) -> ("error out"=w461:errorcluster)  [unwired: 5 in, 1 out]
      n180 = invoke class="VI" method="FP.Close"(error in=w461) -> ()  [unwired: 2 in, 3 out]
    }
  }
  n181 = call <vilib>:"Clear Errors.vi"("error in (no error)"=w14) -> ("error out"=w13:errorcluster)  [unwired: 5 in, 1 out]
  n182 = call "TAT_LABVIEW_TO_PLC.vi"("Enum"=enum16{"Read", "Write"}."Read", "error in (no error)"=w19) -> ("error out"=w22:errorcluster, "Array 2"=w23:bool[])  [unwired: 8 in]
  n183 = call <vilib>:"DB Tools Close Connection.vi"("error in (no error)"=w13, "connection reference"=w12) -> ()  [unwired: 5 in, 1 out]
  n184 = Insert Into Array(array=w23, new element=TRUE ("new element/subarray")) -> (w24:bool[])  [unwired: 1 in]
  n185 = call "TAT_LABVIEW_TO_PLC.vi"("Enum"=enum16{"Read", "Write"}."Write", "error in (no error)"=w22, "Array"=w24) -> ()  [unwired: 7 in, 2 out]
  "CYCLE STATUS STATION 1" <- ""
  "QR STATION 1" <- ""
  "RESULT STATION 1" <- FALSE ("want seconds? (F)")
